vi "Write TaskDAQmx.vi"(8 "error in (no error)":errorcluster, 10 "TaskDAQmx":refnum<k21>, 11 "NiBase in":refnum<class "NiBase.lvclass">) -> (0 "error out":errorcluster, 3 "NiBase out":refnum<class "NiBase.lvclass">)   [LabVIEW 2014, in "FGenPlugins.lvlib" / "NiBase.lvclass"]
uses:
  NiBase.lvclass
  NiBase.lvclass/NiBase.ctl
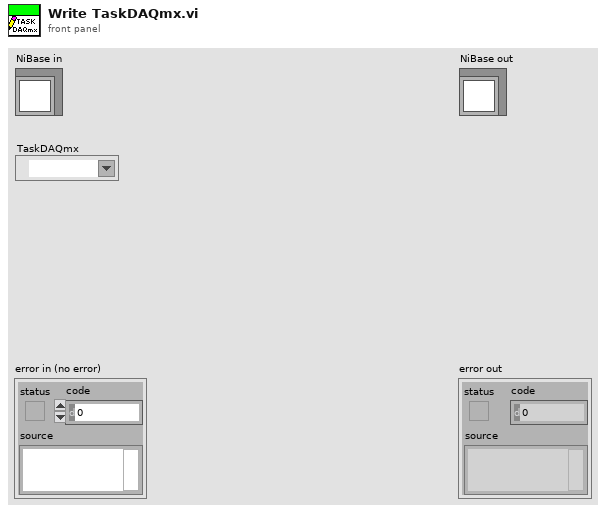
[diagram p1: front panel]
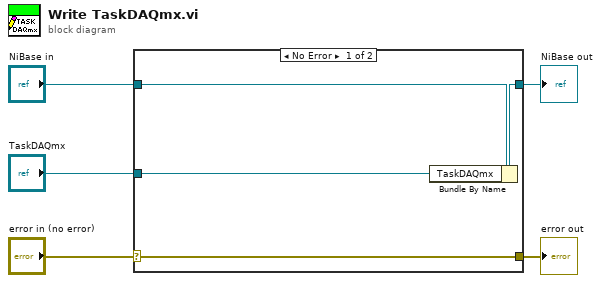
[diagram p0: block diagram]
diagram:
  n1 = case shown="No Error" "error in (no error)" {
    selector: "error in (no error)" -> [w9 w10]
    tunnel: [w9 w10] -> w4
    tunnel: [w7 w11] -> w2
    tunnel: "NiBase in" -> [w8 w11]
    tunnel: "TaskDAQmx" -> [w6 _]
    frame No Error {
      n2 = Bundle By Name(cluster=w8, "TaskDAQmx"=w6) -> (w7:refnum<class "NiBase.lvclass">)
    }
    frame Error {
    }
  }
  "error out" <- w4
  "NiBase out" <- w2
